vi "Add Model.vi"(7 "Overwrite Existing?":bool=TRUE, 8 "error in (no error)":errorcluster, 9 "Settings":T1, 10 "Base Node Path":string, 11 "SysDef Ref":T2) -> (0 "error out":errorcluster, 2 "New Node Path":string, 3 "SysDef Ref Out":T2)   [LabVIEW 2019, in "Simple SysDef API.lvlib"]
uses:
  <userlib>/SimpleSysDef/Simple SysDef API.lvlib
  <userlib>/SimpleSysDef/_SubVIs/System Definition Reference.ctl
  NationalInstruments.VeriStand.SystemDefinitionAPI
  <userlib>/SimpleSysDef/_SubVIs/Add Model_Settings.ctl
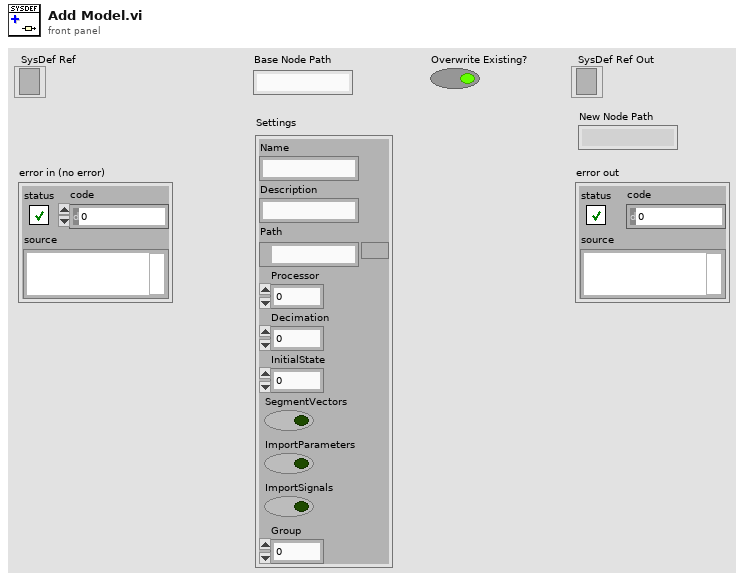
[diagram p1: front panel]
types:
  T1 = typedef "Simple SysDef API.lvlib/Add Model_Settings.ctl" = cluster{"Name":string, "Description":string, "Path":path, "Processor":i32, "Decimation":i32, "InitialState":u16, "SegmentVectors":bool, "ImportParameters":bool, "ImportSignals":bool, "Group":i32}
  T2 = typedef "Simple SysDef API.lvlib/System Definition Reference.ctl" = refnum<k24>
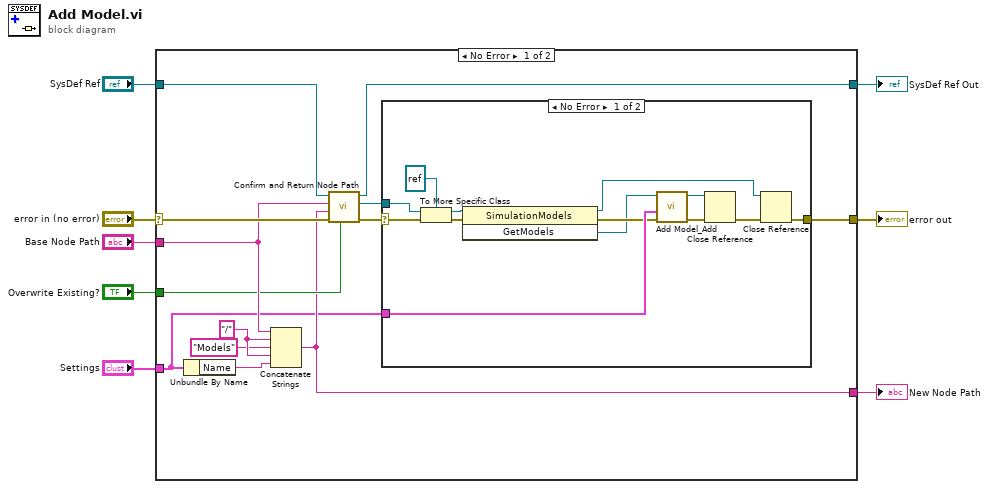
[diagram p0: block diagram]
diagram:
  n1 = case shown="No Error" "error in (no error)" {
    selector: "error in (no error)" -> [w21 w37]
    tunnel: [w17 w37] -> w7
    tunnel: "SysDef Ref" -> [w20 w36]
    tunnel: [w19 w36] -> w5
    tunnel: "Base Node Path" -> [w14 _]
    tunnel: "Overwrite Existing?" -> [w13 _]
    tunnel: "Settings" -> [w11 _]
    tunnel: [w12 _] -> w1
    frame No Error {
      w10 = "/" ("string")
      n2 = Unbundle By Name(w11) -> ("Name"=w18:string)
      n3 = Concatenate Strings(w14, w10, "Models" ("string"), w10, w18) -> (w12:string)
      n4 = call <userlib>:"Confirm and Return Node Path.vi"("Overwrite Existing?"=w13, "error in (no error)"=w21, "New Node Path"=w12, "Base Node Path"=w14, "SysDef Ref"=w20) -> ("error out"=w15:errorcluster, "Node Ref"=w16:refnum<k24>, "SysDef Ref Out"=w19:T2)  [unwired: 4 in]
      n5 = case shown="No Error" w15 {
        selector: w15 -> [w33 w35]
        tunnel: [w25 w35] -> w17
        tunnel: w16 -> [w34 _]
        tunnel: w11 -> [w29 _]
        frame No Error {
          n6 = To More Specific Class(target class=refnum<k24> refnum ("Node Ref"), reference=w34, error in=w33) -> (specific class reference=w23:refnum<k24>, error out=w28:errorcluster)
          n7 = invoke class="SimulationModels" method="GetModels"(reference=w23, error in=w28) -> (reference out=w24:refnum<k24>, error out=w27:errorcluster, "GetModels"=w22:refnum<k24>)  [unwired: 1 in]
          n8 = call <userlib>:"Add Model_Add.vi"("error in (no error)"=w27, "Settings"=w29, "Model Ref"=w22) -> ("error out"=w31:errorcluster, "Model Ref Out"=w30:refnum<k24>)  [unwired: 7 in]
          n9 = Close Reference(reference=w30, error in (no error)=w31) -> (error out=w26:errorcluster)
          n10 = Close Reference(reference=w24, error in (no error)=w26) -> (error out=w25:errorcluster)
        }
        frame Error {
        }
      }
    }
    frame Error {
    }
  }
  "SysDef Ref Out" <- w5
  "error out" <- w7
  "New Node Path" <- w1
